vi "Get Connection Properties.vi"(8 "error in (no error)":errorcluster, 11 "Device Item Ref in":T1 format="%.0x") -> (0 "error out":errorcluster, 2 "AutoSelect":T2, 3 "Item Ref out":T1 format="%.0x")   [LabVIEW 2017, in "Chassis TimeSync System Explorer.lvlib"]
uses:
  Chassis TimeSync System Explorer.lvlib
  Shared/Connection Settings.ctl
  Shared/Mode.ctl
  Shared/External Pin.ctl
  Shared/Routes.ctl
  Shared/Route.ctl
  <vilib>/NI Veristand/Custom Device API/Custom Device Item Ref.ctl
  Shared/Constants.vi
  <vilib>/NI Veristand/Custom Device API/Get Item Property (U16).vi
  <vilib>/NI Veristand/Custom Device API/Get Item Property (Boolean).vi
  Shared/Chassis TimeSync Shared.lvlib
  <vilib>/NI Veristand/Custom Device API/Custom Device API.lvlib
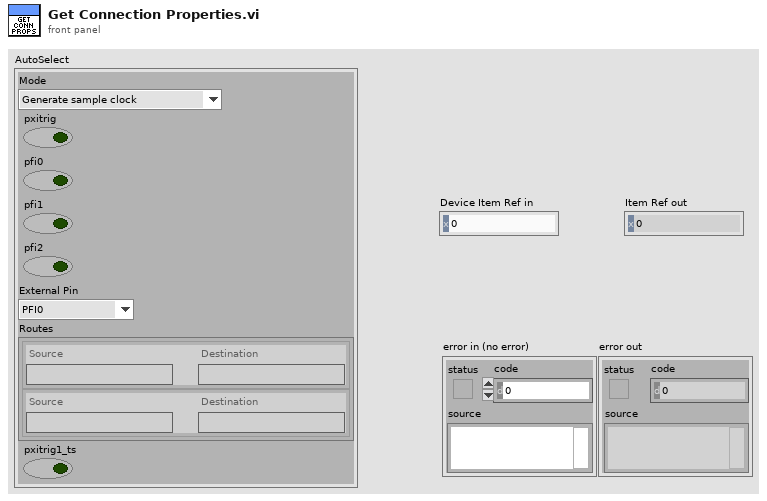
[diagram p1: front panel]
types:
  T1 = typedef "Custom Device API.lvlib/Custom Device Item Ref.ctl" = u64
  T2 = typedef "Chassis TimeSync Shared.lvlib/Connection Settings.ctl" = cluster{"Mode":T3, "pxitrig":bool, "pfi0":bool, "pfi1":bool, "pfi2":bool, "External Pin":T4, "Routes":T5, "pxitrig1_ts":bool}
  T3 = typedef "Chassis TimeSync Shared.lvlib/Mode.ctl" = enum16{"Generate sample clock", "Route sample clock out of chassis", "Route sample clock into chassis", "Custom routes"}
  T4 = typedef "Chassis TimeSync Shared.lvlib/External Pin.ctl" = enum16{"PFI0", "PFI1", "PFI2"}
  T5 = typedef "Chassis TimeSync Shared.lvlib/Routes.ctl" = T6[]
  T6 = typedef "Chassis TimeSync Shared.lvlib/Route.ctl" = cluster{"Source":string, "Destination":string}
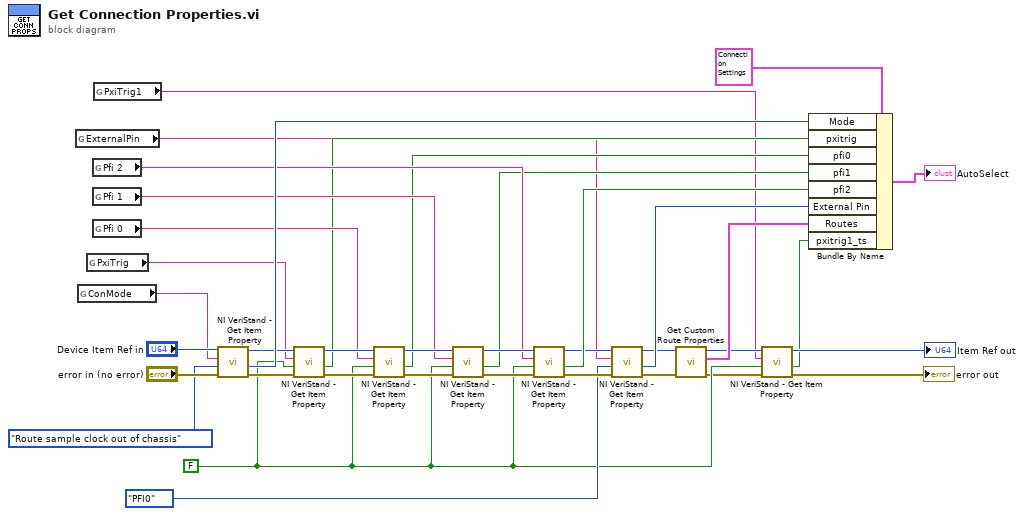
[diagram p0: block diagram]
diagram:
  w7 = FALSE ("pxitrig")
  n1 = global read "Constants.vi" "ExternalPin"() -> (w13:string)
  n2 = global read "Constants.vi" "ConMode"() -> (w34:string)
  n3 = global read "Constants.vi" "PxiTrig"() -> (w29:string)
  n4 = global read "Constants.vi" "Pfi 2"() -> (w20:string)
  n5 = global read "Constants.vi" "Pfi 1"() -> (w23:string)
  n6 = global read "Constants.vi" "Pfi 0"() -> (w26:string)
  n7 = global read "Constants.vi" "PxiTrig1"() -> (w2:string)
  n8 = call-poly <vilib>:"NI VeriStand - Get Item Property.vi"("error in (no error)"="error in (no error)", "Default Value"=Mode."Route sample clock out of chassis" ("Mode"), "Property Name"=w34, "Item Ref in"="Device Item Ref in") -> ("error out"=w30:errorcluster, "Value"=w32:u16, "Item Ref out"=w31:T1)  [unwired: 4 in, 1 out]
  n9 = call-poly <vilib>:"NI VeriStand - Get Item Property.vi"("error in (no error)"=w30, "Default Value"=w7, "Property Name"=w29, "Item Ref in"=w31) -> ("error out"=w27:errorcluster, "Value"=w19:bool, "Item Ref out"=w28:T1)  [unwired: 4 in, 1 out]
  n10 = call-poly <vilib>:"NI VeriStand - Get Item Property.vi"("error in (no error)"=w27, "Default Value"=w7, "Property Name"=w26, "Item Ref in"=w28) -> ("error out"=w24:errorcluster, "Value"=w18:bool, "Item Ref out"=w25:T1)  [unwired: 4 in, 1 out]
  n11 = call-poly <vilib>:"NI VeriStand - Get Item Property.vi"("error in (no error)"=w24, "Default Value"=w7, "Property Name"=w23, "Item Ref in"=w25) -> ("error out"=w21:errorcluster, "Value"=w17:bool, "Item Ref out"=w22:T1)  [unwired: 4 in, 1 out]
  n12 = call-poly <vilib>:"NI VeriStand - Get Item Property.vi"("error in (no error)"=w21, "Default Value"=w7, "Property Name"=w20, "Item Ref in"=w22) -> ("error out"=w15:errorcluster, "Value"=w16:bool, "Item Ref out"=w14:T1)  [unwired: 4 in, 1 out]
  n13 = call-poly <vilib>:"NI VeriStand - Get Item Property.vi"("error in (no error)"=w15, "Default Value"=External_Pin."PFI0" ("External Pin"), "Property Name"=w13, "Item Ref in"=w14) -> ("error out"=w10:errorcluster, "Value"=w11:u16, "Item Ref out"=w9:T1)  [unwired: 4 in, 1 out]
  n14 = call "Get Custom Route Properties.vi"("error in (no error)"=w10, "Item Ref in"=w9) -> ("error out"=w5:errorcluster, "Routes"=w8:T5, "Item Ref out"=w6:T1)  [unwired: 7 in]
  n15 = call-poly <vilib>:"NI VeriStand - Get Item Property.vi"("error in (no error)"=w5, "Default Value"=w7, "Property Name"=w2, "Item Ref in"=w6) -> ("error out"=→"error out":errorcluster, "Value"=w1:bool, "Item Ref out"=→"Item Ref out":T1)  [unwired: 4 in, 1 out]
  n16 = Bundle By Name(cluster=T2 {"Mode"=enum."Generate sample clock", "pxitrig"=FALSE, "pfi0"=TRUE, "pfi1"=TRUE, "pfi2"=TRUE, "External Pin"=enum."PFI0", "Routes"=[], "pxitrig1_ts"=FALSE}, "Mode"=w32, "pxitrig"=w19, "pfi0"=w18, "pfi1"=w17, "pfi2"=w16, "External Pin"=w11, "Routes"=w8, "pxitrig1_ts"=w1) -> (→"AutoSelect":T2)
